vi "CRCStream.vi"(1 "Data":u8, 2 "Numeric in":u16) -> (0 "Numeric out":u16)   [LabVIEW 2018, in "Modbus_Processing_Unit.lvlib"]
uses:
  Modbus_Processing_Unit.lvlib
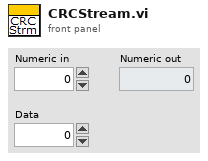
[diagram p1: front panel]
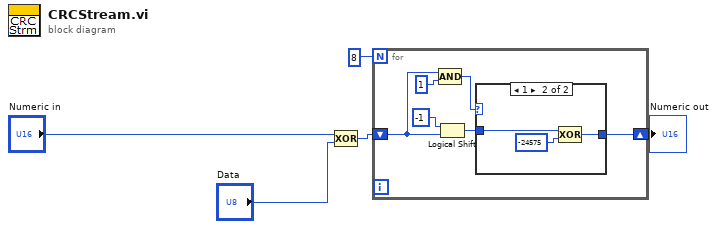
[diagram p0: block diagram]
diagram:
  n1 = Compound Arithmetic op=XOR("Numeric in", "Data") -> (w3:u16)
  n2 = for {
    N: i16 8 -> [_]
    shift-right: [w8] -> w4
    shift-left: w3 -> [w9]
    n3 = Logical Shift(y=i16 -1, x=w9) -> (x << y=w6:u16)
    n4 = Compound Arithmetic op=AND(w9, i16 1) -> (w11:u16)
    n5 = case shown="1" w11 {
      tunnel: [w12 w15] -> w8
      tunnel: w6 -> [w12 w13]
      frame 0, Default {
      }
      frame 1 {
        n6 = Compound Arithmetic op=XOR(w13, i16 -24575) -> (w15:u16)
      }
    }
  }
  "Numeric out" <- w4
